vi "UpdateControlsFromMCListbox.vi"(8 "error in (no error)":errorcluster, 10 "MulticolumnListbox in":refnum<vi>, 11 "Controls in":T1[](array[typedef])) -> (0 "error out":errorcluster, 3 "Controls out":T1[](array[typedef]))   [LabVIEW 2017, in "ContextHelpEditor.lvlib"]
uses:
  ContextHelpEditor.lvlib
  ControlRef--cluster.ctl
  <vilib>/picture/picture.llb/imagedata.ctl
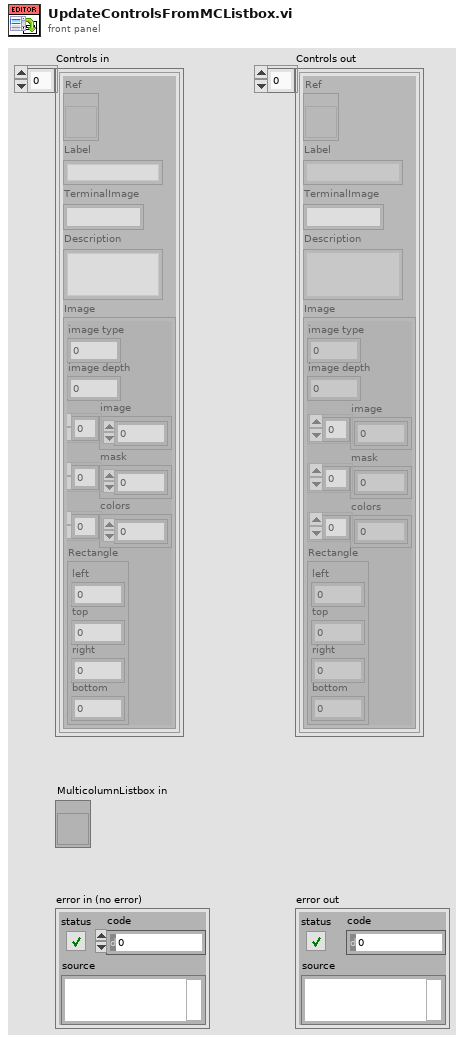
[diagram p1: front panel]
types:
  T1 = typedef "ContextHelpEditor.lvlib/ControlRef--cluster.ctl" = cluster{"Ref":refnum<vi>, "Label":string, "TerminalImage":picture, "Description":string, "Image":T2}
  T2 = typedef "imagedata.ctl" = cluster{"image type":i32, "image depth":i32, "image":u8[], "mask":u8[], "colors":u32[], "Rectangle":cluster{"left":i16, "top":i16, "right":i16, "bottom":i16}}
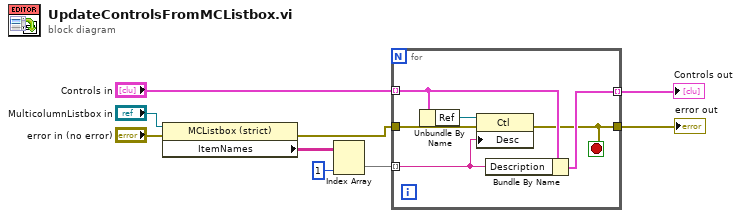
[diagram p0: block diagram]
diagram:
  n1 = property class="MCListbox (strict)"(reference="MulticolumnListbox in", error in="error in (no error)") -> (error out=w8:errorcluster, "ItemNames"=w5:string[][])  [unwired: 1 out]
  n2 = Index Array(array=w5, index (col)=1 ("disabled index (col)")) -> (element=w7:string[])  [unwired: 1 in]
  n3 = for {
    tunnel: "Controls in" -> [w14] mode=indexing
    tunnel: [w15] -> w2 mode=indexing
    tunnel: w8 -> [w12]
    tunnel: [w11] -> w3
    tunnel: w7 -> [w10] mode=indexing
    stop <- w11 stop-if-true
    n4 = Unbundle By Name(w14) -> ("Ref"=w13:refnum<vi>)
    n5 = property class="Ctl"(reference=w13, error in=w12, "Desc"=w10) -> (error out=w11:errorcluster)  [unwired: 1 out]
    n6 = Bundle By Name(cluster=w14, "Description"=w10) -> (w15:T1)
  }
  "error out" <- w3
  "Controls out" <- w2
